vi "Data Tag.vi"(8 "error in (no error)":errorcluster, 11 "Node Ptr":T1 format="%.0x") -> (0 "error out":errorcluster)   [LabVIEW 2013, in "OPC UA Client System Explorer.lvlib"]
uses:
  OPC UA Client System Explorer.lvlib
  <vilib>/NI Veristand/Custom Device API/Custom Device Item Ref.ctl
  Shared/Constants.vi
  <vilib>/NI Veristand/Custom Device API/Get Item Property (U32).vi
  <vilib>/NI Veristand/Custom Device API/Get Item Property (String).vi
  <vilib>/NI Veristand/Custom Device API/Custom Device API.lvlib
  Shared/OPC UA Client Shared.lvlib
panel:
  out "DataType":u32(ring)=1 items=["Boolean"=1, "SByte"=2, "Byte"=3, "Int16"=4, "UInt16"=5, "Int32"=6, "UInt32"=7, "Int64"=8, "UInt64"=9, "Float"=10, "Double"=11, "String"=12, "DateTime"=13, "ByteString"=15, "Array of Boolean"=101, "Array of SByte"=102, "Array of Byte"=103, "Array of Int16"=104, "Array of UInt16"=105, "Array of Int32"=106, "Array of UInt32"=107, "Array of Int64"=108, "Array of UInt64"=109, "Array of Float"=110, "Array of Double"=111, "Array of String"=112, "Array of DateTime"=113, "Array of ByteString"=115]
  out "Tag Path":string
  out "Name":string
  in  "Header":cluster{"Section Name":string}={"Section Name"="Data Tag Settings"}
  in  "SHDocVw.IWebBrowser":refnum<k7>(container)
  in  "Description":string
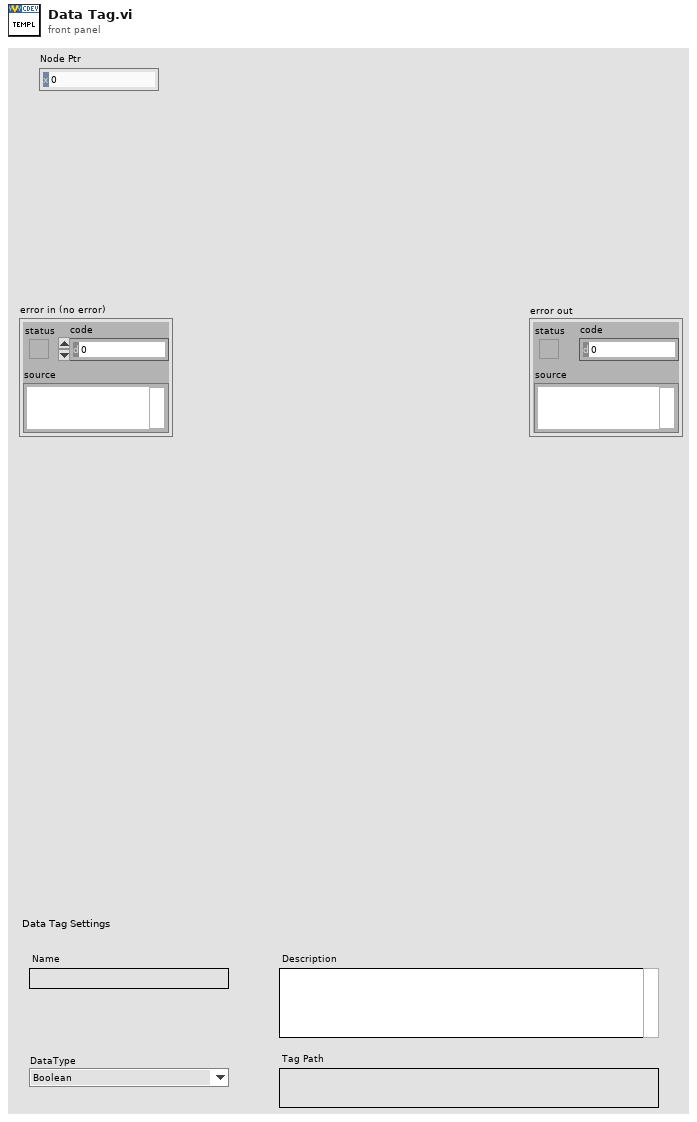
[diagram p1: front panel]
types:
  T1 = typedef "Custom Device API.lvlib/Custom Device Item Ref.ctl" = u64
  T2 = typedef "Custom Device API.lvlib/Custom Device Item Info.ctl" = cluster{"Name":string, "Is Channel":bool, "GUID":string, "Is Waveform":bool}
  T3 = typedef "Custom Device API.lvlib/Custom Device Commands.ctl" = enum16{"Default", "Item renamed", "Shutdown", "Dynamic button pressed"}
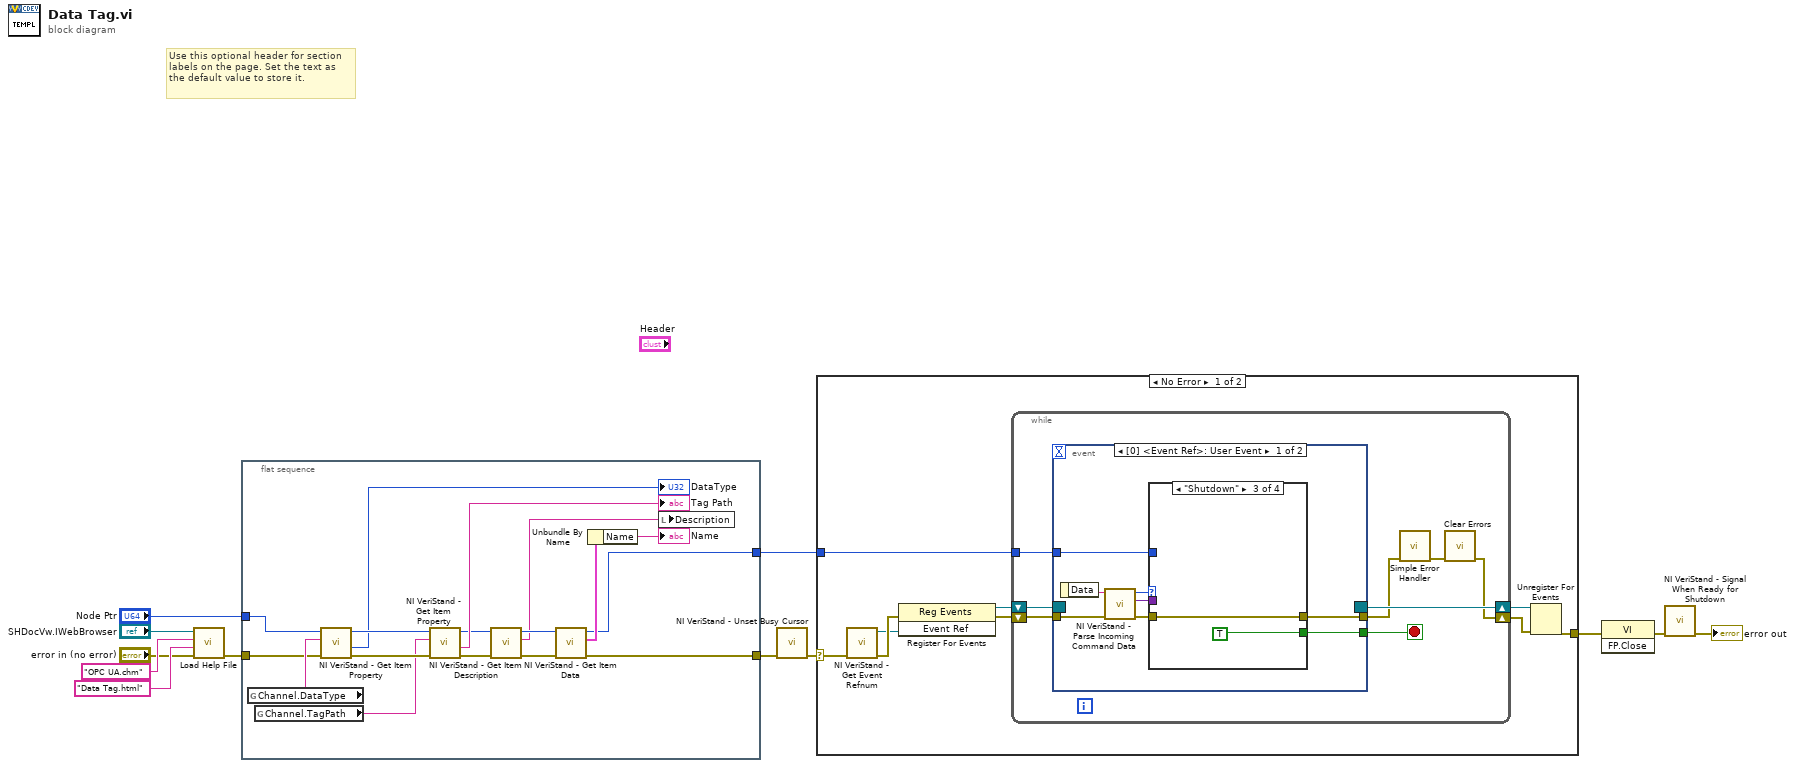
[diagram p0: block diagram]
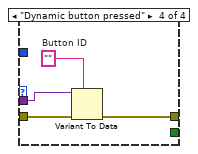
[diagram p4: hidden frame]
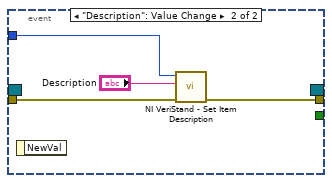
[diagram p5: hidden frame]
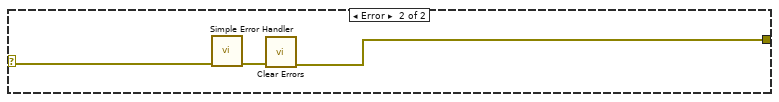
[diagram p6: hidden frame]
diagram:
  # "Use this optional header for section labels on the page. Set the text as the default value to store it."
  n1 = call "Load Help File.vi"("error in (no error)"="error in (no error)", "HTML File"="Data Tag.html" ("Main CHM File"), "Main CHM File"="OPC UA.chm", "SHDocVw.IWebBrowser2"="SHDocVw.IWebBrowser") -> ("error out"=w3:errorcluster)  [unwired: 7 in]
  n2 = flat-sequence {
    tunnel: "Node Ptr" -> [w23]
    tunnel: w3 -> [w22]
    tunnel: [w17] -> w2
    tunnel: [w15] -> w1
    frame #0 {
      n3 = global read "Constants.vi" "Channel.DataType"() -> (w27:string)
      n4 = global read "Constants.vi" "Channel.TagPath"() -> (w26:string)
      n5 = call-poly <vilib>:"NI VeriStand - Get Item Property.vi"("error in (no error)"=w22, "Property Name"=w27, "Item Ref in"=w23) -> ("error out"=w28:errorcluster, "Value"=→"DataType":u32, "Item Ref out"=w29:T1)  [unwired: 5 in, 1 out]
      n6 = call-poly <vilib>:"NI VeriStand - Get Item Property.vi"("error in (no error)"=w28, "Property Name"=w26, "Item Ref in"=w29) -> ("error out"=w21:errorcluster, "Value"=→"Tag Path":string, "Item Ref out"=w20:T1)  [unwired: 5 in, 1 out]
      n7 = call <vilib>:"NI VeriStand - Get Item Description.vi"("error in (no error)"=w21, "Item Ref in"=w20) -> ("error out"=w18:errorcluster, "Description"=w13:string, "Item Ref out"=w16:T1)  [unwired: 6 in, 1 out]
      n8 = call <vilib>:"NI VeriStand - Get Item Data.vi"("error in (no error)"=w18, "Item Ref in"=w16) -> ("error out"=w17:errorcluster, "Item Info"=w19:T2, "Item Ref out"=w15:T1)  [unwired: 7 out]
      n9 = Unbundle By Name(w19) -> ("Name"=→"Name":string)
      n10 = local write "Description"(w13) -> ()
    }
  }
  n11 = call <vilib>:"NI VeriStand - Unset Busy Cursor.vi"("error in (no error)"=w2) -> ("error out"=w9:errorcluster)  [unwired: 10 out]
  n12 = case shown="No Error" w9 {
    selector: w9 -> [w30 w69]
    tunnel: [w35 w67] -> w12
    tunnel: w1 -> [w31 _]
    frame No Error {
      n13 = call <vilib>:"NI VeriStand - Get Event Refnum.vi"("error in (no error)"=w30) -> ("error out"=w38:errorcluster, "Event Ref"=w34:refnum<user-event>)  [unwired: 9 out]
      n14 = register-events(error in=w38, w34) -> (reference out=w32:refnum<event-registration>, error out=w33:errorcluster)  [unwired: 1 in]
      n15 = while {
        tunnel: w31 -> [w42]
        shift-right: [w39] -> w36
        shift-left: w33 -> [w45]
        shift-right: [w46] -> w37
        shift-left: w32 -> [w44]
        stop <- w43 stop-if-true
        n16 = event shown="[0] <Event Ref>: User Event" {
          selector: w44 -> [_ _]
          dyn-events: [_ _] -> w46
          timeout: _ -> [_ _]
          tunnel: w45 -> [w54 w66]
          tunnel: [w50 _] -> w43
          tunnel: [w49 w64] -> w41
          tunnel: w42 -> [w48 w65]
          event User Event {
            n17 = event-data() -> ("Data"=w53:string)  [unwired: 1 out]
            n18 = call <vilib>:"NI VeriStand - Parse Incoming Command Data.vi"("error in (no error)"=w54, "Incoming data"=w53) -> ("error out"=w52:errorcluster, "Outgoing data"=w47:variant, "Action"=w51:T3)  [unwired: 7 out]
            n19 = case shown="\"Shutdown\"" w51 {
              tunnel: w52 -> [w55 w56 w57 w62]
              tunnel: [_ _ TRUE _] -> w50
              tunnel: [w55 w56 w57 w59] -> w49
              tunnel: w48 -> [_ _ _ _]
              tunnel: w47 -> [_ _ _ w61]
              frame "Default", Default {
              }
              frame "Item renamed" {
              }
              frame "Shutdown" {
              }
              frame "Dynamic button pressed" {
                w60 = ""  # Button ID
                n20 = Variant To Data(error in=w62, type=w60, Variant=w61) -> (error out=w59:errorcluster)  [unwired: 1 out]
              }
            }
          }
          event "Description": Value Change {
            n21 = event-data() -> ()  [unwired: 2 out]
            n22 = call <vilib>:"NI VeriStand - Set Item Description.vi"("error in (no error)"=w66, "Description"="Description", "Item Ref in"=w65) -> ("error out"=w64:errorcluster)  [unwired: 6 in, 2 out]
          }
        }
        n23 = call <vilib>:"Simple Error Handler.vi"("error in (no error)"=w41) -> ("error out"=w40:errorcluster)  [unwired: 1 in, 7 out]
        n24 = call <vilib>:"Clear Errors.vi"("error in (no error)"=w40) -> ("error out"=w39:errorcluster)  [unwired: 6 out]
      }
      n25 = Unregister For Events(event registration refnum=w37, error in=w36) -> (error out=w35:errorcluster)
    }
    frame Error {
      n26 = call <vilib>:"Simple Error Handler.vi"("error in (no error)"=w69) -> ("error out"=w68:errorcluster)  [unwired: 1 in, 7 out]
      n27 = call <vilib>:"Clear Errors.vi"("error in (no error)"=w68) -> ("error out"=w67:errorcluster)  [unwired: 6 out]
    }
  }
  n28 = invoke class="VI" method="FP.Close"(error in=w12) -> (error out=w11:errorcluster)  [unwired: 2 in, 2 out]
  n29 = call <vilib>:"NI VeriStand - Signal When Ready for Shutdown.vi"("error in (no error)"=w11) -> ("error out"=→"error out":errorcluster)  [unwired: 10 out]
